vi "Set Control Labels.vi"(8 "error in (no error)":errorcluster, 10 "Display State In 2":T1={"Show Axes"=FALSE, "Show Y=0"=FALSE, "Controls"={"Type"=enum."Sine", "Periods"=0.0, "Points"=0, "Offset"=0.0, "Amplitdue"=0.0, "Starting Phase"=0.0, "func"=""}, "Show Current Location"=FALSE, "Current Location"=0, "dt"=0.0, "t0"=timestamp(0 s since 1904-01-01), "Amplitude Format String"="%_3p"} caption="State" {"Controls"."Points" format="%_3p"}, 11 "Controlst":refnum<vi>) -> (0 "error out":errorcluster, 2 "Display State Out":T1={"Show Axes"=FALSE, "Show Y=0"=FALSE, "Controls"={"Type"=enum."Sine", "Periods"=0.0, "Points"=0, "Offset"=0.0, "Amplitdue"=0.0, "Starting Phase"=0.0, "func"=""}, "Show Current Location"=FALSE, "Current Location"=0, "dt"=0.0, "t0"=timestamp(0 s since 1904-01-01), "Amplitude Format String"="%_3p"} caption="State" {"Controls"."Points" format="%_3p"})   [LabVIEW 2012]
uses:
  Controls/Waveform State.ctl
  FP Controls.ctl
  Function Types.ctl
  Waveform Control.xctl
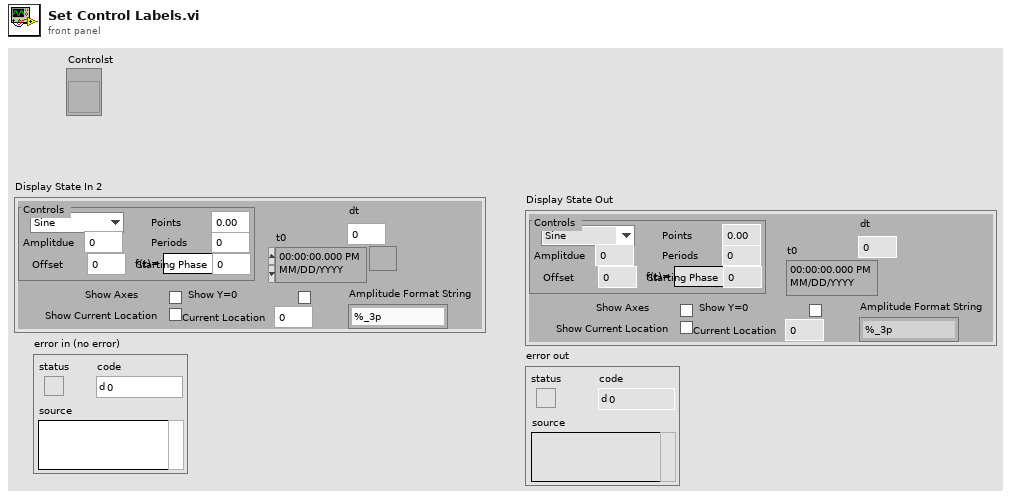
[diagram p1: front panel]
types:
  T1 = typedef "Waveform Control.xctl/Waveform State.ctl" = cluster{"Show Axes":bool, "Show Y=0":bool, "Controls":T2, "Show Current Location":bool, "Current Location":i32, "dt":dbl, "t0":timestamp, "Amplitude Format String":string}
  T2 = typedef "Waveform Control.xctl/FP Controls.ctl" = cluster{"Type":T3, "Periods":dbl, "Points":i32, "Offset":dbl, "Amplitdue":dbl, "Starting Phase":dbl, "func":string}
  T3 = typedef "Waveform Control.xctl/Function Types.ctl" = enum16{"Level", "Sine", "Triangle", "Ramp", "Saw Tooth", "Square", "Function"}
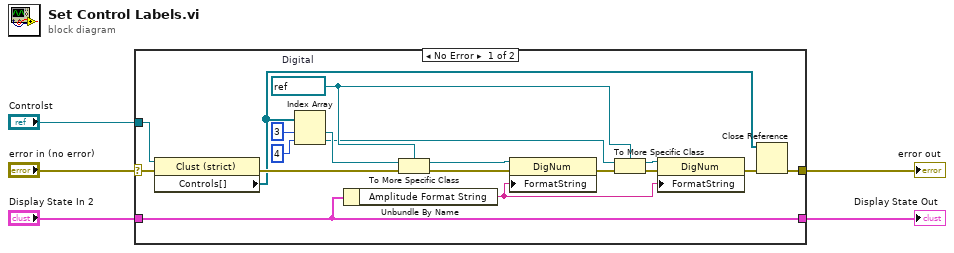
[diagram p0: block diagram]
diagram:
  n1 = case shown="No Error" "error in (no error)" {
    selector: "error in (no error)" -> [w22 w24]
    tunnel: "Display State In 2" -> [w6 w25]
    tunnel: "Controlst" -> [w23 _]
    tunnel: [w7 w24] -> w2
    tunnel: [w6 w25] -> w1
    frame No Error {
      w15 = refnum<vi> refnum  # Digital
      n2 = property class="Clust (strict)"(reference=w23, error in=w22) -> (error out=w17:errorcluster, "Controls[]"=w8:refnum<vi>[])  [unwired: 1 out]
      n3 = Index Array(array=w8, index #1=3 ("index"), index #2=4 ("index")) -> (element #1=w19:refnum<vi>, element #2=w14:refnum<vi>)
      n4 = Unbundle By Name(w6) -> ("Amplitude Format String"=w10:string)
      n5 = To More Specific Class(target class=w15, reference=w19, error in=w17) -> (specific class reference=w18:refnum<vi>, error out=w16:errorcluster)
      n6 = property class="DigNum"(reference=w18, error in=w16, "FormatString"=w10) -> (error out=w13:errorcluster)  [unwired: 1 out]
      n7 = To More Specific Class(target class=w15, reference=w14, error in=w13) -> (specific class reference=w11:refnum<vi>, error out=w12:errorcluster)
      n8 = property class="DigNum"(reference=w11, error in=w12, "FormatString"=w10) -> (error out=w9:errorcluster)  [unwired: 1 out]
      n9 = Close Reference(reference=w8, error in (no error)=w9) -> (error out=w7:errorcluster)
    }
    frame Error {
    }
  }
  "Display State Out" <- w1
  "error out" <- w2
